vi "HMI Command (array).vi"(9 "RIO CMD":dbl[](array[numeric])=[0.0, 0.0, 0.0, 0.0, 0.0, 0.0] min=0.0 max=100.0 step=0.1 format="%#.2f", 10 "HMI CMD":dbl[](array[numeric]), 11 "Prev CMD":dbl[](array[numeric])) -> (2 "Boolean":bool, 3 "CMD OUT":dbl[](array[numeric]))   [LabVIEW 2019]
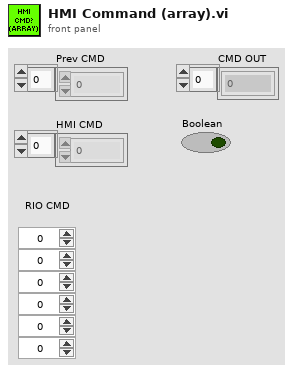
[diagram p1: front panel]
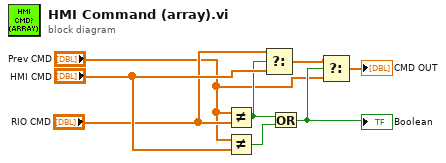
[diagram p0: block diagram]
diagram:
  n1 = Not Equal?(x="Prev CMD", y="RIO CMD") -> (x != y?=w6:bool)
  n2 = Not Equal?(x="Prev CMD", y="HMI CMD") -> (x != y?=w5:bool)
  n3 = Select(t="RIO CMD", s=w6, f="HMI CMD") -> (s? t:f=w3:dbl[])
  n4 = Or(x=w6, y=w5) -> (x .or. y?=w4:bool)
  "Boolean" <- w4
  n5 = Select(t=w3, s=w4, f="Prev CMD") -> (s? t:f=→"CMD OUT":dbl[])
